vi "图像位移2振镜偏转角.vi"(8 "图像位移(um)":dbl[](array[numeric]), 9 "f_objecitve(mm)":dbl=1.8, 10 "f_tubelens(mm)":dbl=200.0, 11 "f_scanlens(mm)":dbl=50.0) -> (0 "振镜偏转角(°)":dbl[](array[numeric]))   [LabVIEW 2015]
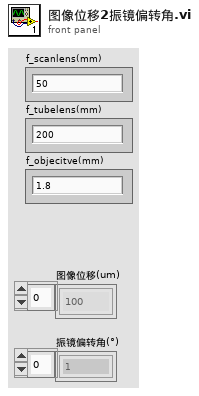
[diagram p1: front panel]
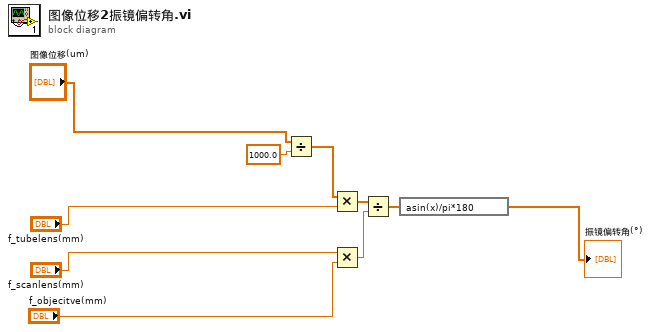
[diagram p0: block diagram]
diagram:
  n1 = Divide(x="图像位移(um)", y=1000.0) -> (x/y=w6:dbl[])
  n2 = Multiply(x=w6, y="f_tubelens(mm)") -> (x*y=w10:dbl[])
  n3 = Multiply(x="f_scanlens(mm)", y="f_objecitve(mm)") -> (x*y=w9:dbl)
  n4 = Divide(x=w10, y=w9) -> (x/y=w8:dbl[])
  n5 = expression code="asin(x)/pi*180"(w8) -> (→"振镜偏转角(°)":dbl[])
